vi "F4.vi"(8 "s":dbl, 9 "d":dbl, 10 "w":dbl, 11 "a":dbl) -> (2 "F4":dbl format="%#_13g")   [LabVIEW 2021]
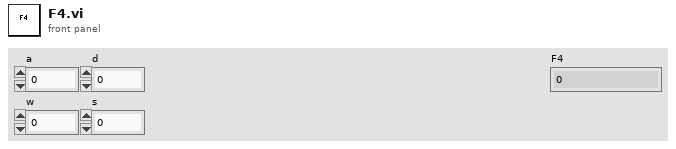
[diagram p1: front panel]
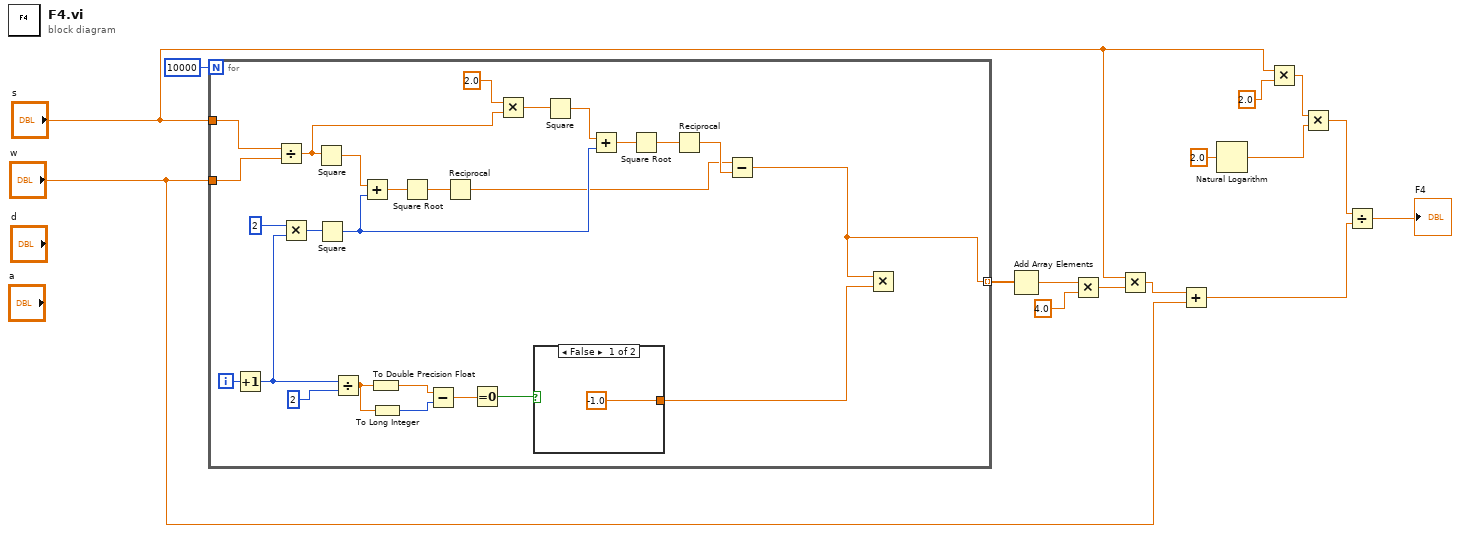
[diagram p0: block diagram]
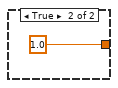
[diagram p2: hidden frame]
diagram:
  n1 = for {
    N: 10000 -> [_]
    tunnel: "s" -> [w40]
    tunnel: "w" -> [w39]
    tunnel: [w20] -> w15 mode=indexing
    i -> [w19]
    n2 = Increment(x=w19) -> (x+1=w18:i32)
    n3 = Divide(x=w40, y=w39) -> (x/y=w28:dbl)
    n4 = Multiply(x=2, y=w18) -> (x*y=w37:i32)
    n5 = Square(x=w28) -> (x^2=w36:dbl)
    n6 = Square(x=w37) -> (x^2=w31:i32)
    n7 = Divide(x=w18, y=2) -> (x/y=w26:dbl)
    n8 = Add(x=w36, y=w31) -> (x+y=w35:dbl)
    n9 = To Double Precision Float(number=w26) -> (double precision float=w25:dbl)
    n10 = To Long Integer(number=w26) -> (32bit integer=w24:i32)
    n11 = Square Root(x=w35) -> (sqrt(x)=w41:dbl)
    n12 = Subtract(x=w25, y=w24) -> (x-y=w23:dbl)
    n13 = Reciprocal(x=w41) -> (1/x=w16:dbl)
    n14 = Equal To 0?(x=w23) -> (x = 0?=w22:bool)
    n15 = Multiply(x=2.0, y=w28) -> (x*y=w30:dbl)
    n16 = case shown="False" w22 {
      tunnel: [-1.0 1.0] -> w21
      frame False {
      }
      frame True {
      }
    }
    n17 = Square(x=w30) -> (x^2=w33:dbl)
    n18 = Add(x=w33, y=w31) -> (x+y=w32:dbl)
    n19 = Square Root(x=w32) -> (sqrt(x)=w34:dbl)
    n20 = Reciprocal(x=w34) -> (1/x=w17:dbl)
    n21 = Subtract(x=w16, y=w17) -> (x-y=w20:dbl)
    n22 = Multiply(x=w20, y=w21) -> ()  [unwired: 1 out]
  }
  n23 = Add Array Elements(numeric array=w15) -> (sum=w14:dbl)
  n24 = Multiply(x=w14, y=4.0) -> (x*y=w12:dbl)
  n25 = Multiply(x="s", y=w12) -> (x*y=w10:dbl)
  n26 = Add(x=w10, y="w") -> (x+y=w2:dbl)
  n27 = Natural Logarithm(1:2.0 ("x")) -> (0:w5:dbl)
  n28 = Multiply(x="s", y=2.0 ("x")) -> (x*y=w6:dbl)
  n29 = Multiply(x=w6, y=w5) -> (x*y=w3:dbl)
  n30 = Divide(x=w3, y=w2) -> (x/y=→"F4":dbl)
